vi "Sensitivity settings.vi"(8 "error in":errorcluster, 11 "Instrument parameters in":T1) -> (0 "error IO":errorcluster, 3 "Instrument parameters out":T1)   [LabVIEW 2025, in "MyLockIn.lvlib"]
uses:
  MyLockIn.lvlib
panel:
  in  "Current pointer":u64=1
  in  "Checking interval":u64=1 min=1 step=1
  in  "Lower limit (%)":dbl
  in  "Upper limit (%)":dbl=100.0
  # "SETTING FOR MONITORING SENSITIVITY"
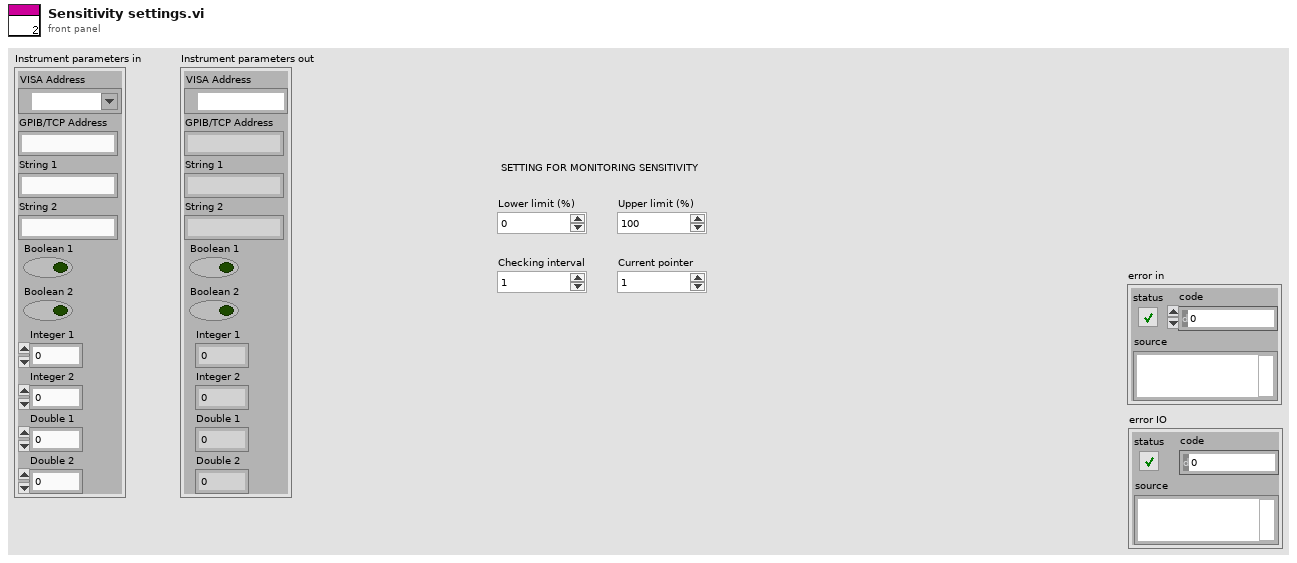
[diagram p1: front panel]
types:
  T1 = cluster{"VISA Address":refnum<visa-resource-name>, "GPIB/TCP Address":string, "String 1":string, "String 2":string, "Boolean 1":bool, "Boolean 2":bool, "Integer 1":i32, "Integer 2":i32, "Double 1":dbl, "Double 2":dbl}
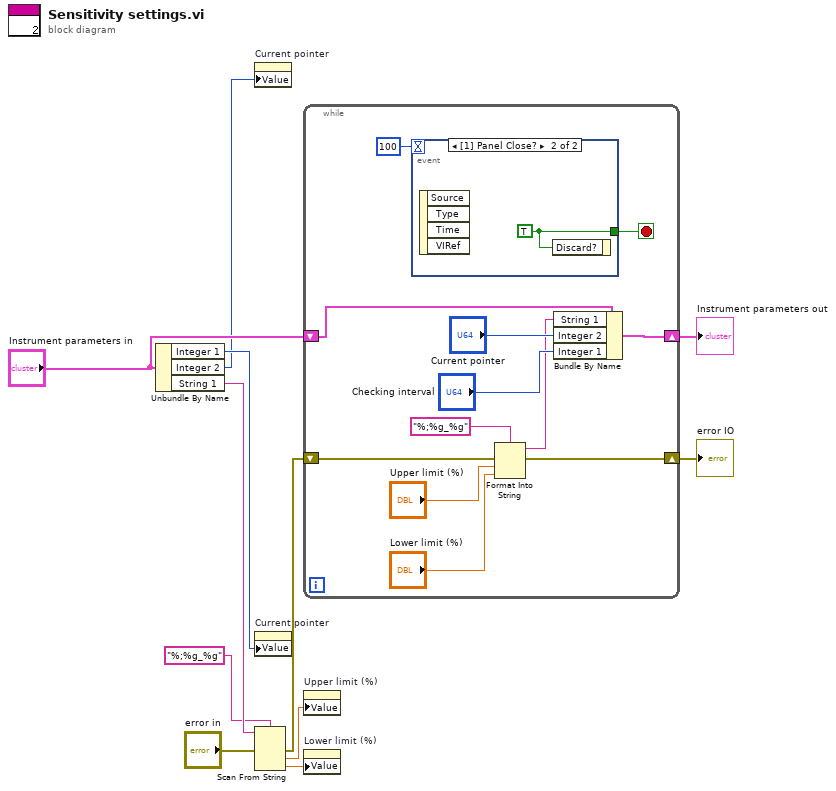
[diagram p0: block diagram]
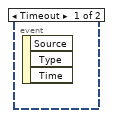
[diagram p2: hidden frame]
diagram:
  n1 = Unbundle By Name("Instrument parameters in") -> ("Integer 1"=w9:i32, "Integer 2"=w8:i32, "String 1"=w7:string)
  n2 = property on="Current pointer" class="DigNum (strict)"("Value"=w8) -> ()  [unwired: 2 in, 2 out]
  n3 = property on="Current pointer" class="DigNum (strict)"("Value"=w9) -> ()  [unwired: 2 in, 2 out]
  n4 = Scan From String(format string="%;%g_%g", input string=w7, error in="error in") -> (error out=w2:errorcluster, output 1=w5:dbl, output 2=w4:dbl)  [unwired: 3 in, 2 out]
  n5 = while {
    shift-right: [w22] -> w11
    shift-left: "Instrument parameters in" -> [w23]
    shift-right: [w12] -> w1
    shift-left: w2 -> [w13]
    stop <- w20 stop-if-true
    n6 = event shown="[1] Panel Close?" {
      selector: _ -> [_ _]
      dyn-events: _ -> [_ _]
      timeout: 100 -> [_ _]
      tunnel: [_ w24] -> w20
      event Timeout {
        n7 = event-data() -> ()  [unwired: 1 in, 3 out]
      }
      event Panel Close? {
        w24 = TRUE ("Discard?")
        n8 = event-data() -> ()  [unwired: 1 in, 4 out]
        n9 = event-data("Discard?"=w24) -> ()  [unwired: 1 in, 1 out]
      }
    }
    n10 = Format Into String(format string="%;%g_%g", error in=w13, "Upper limit (%)", "Lower limit (%)") -> (resulting string=w14:string, error out=w12:errorcluster)  [unwired: 1 in]
    n11 = Bundle By Name(cluster=w23, "String 1"=w14, "Integer 2"="Current pointer", "Integer 1"="Checking interval") -> (w22:T1)
  }
  "Instrument parameters out" <- w11
  "error IO" <- w1
  n12 = property on="Upper limit (%)" class="DigNum (strict)"("Value"=w5) -> ()  [unwired: 2 in, 2 out]
  n13 = property on="Lower limit (%)" class="DigNum (strict)"("Value"=w4) -> ()  [unwired: 2 in, 2 out]
